vi "API - On Demand - Read 1 Digital Input Sample on Demand.vi"(8 "error in":errorcluster, 10 "Digital Input Channel Number":i32, 11 "TCP Network Connection in":refnum<k5>) -> (0 "error out":errorcluster, 2 "Boolean Data Out":bool=TRUE, 3 "TCP Network Connection out":refnum<k5>)   [LabVIEW 2020]
doc: "Read a single digital input measurement from the DAQ.\n-Enable channel\n-Start streaming of data\n-Download 1 datapoint\n-Stop streaming of data"
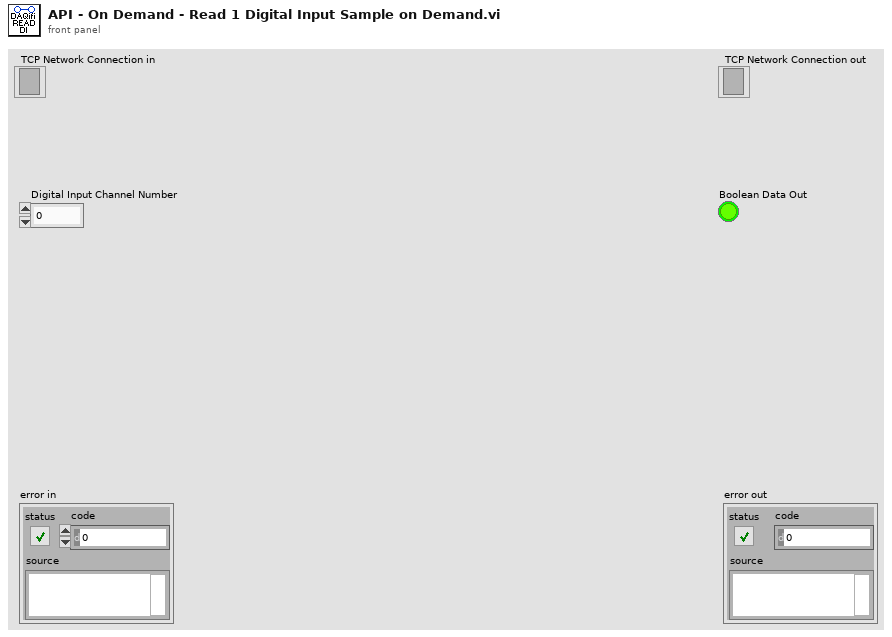
[diagram p1: front panel]
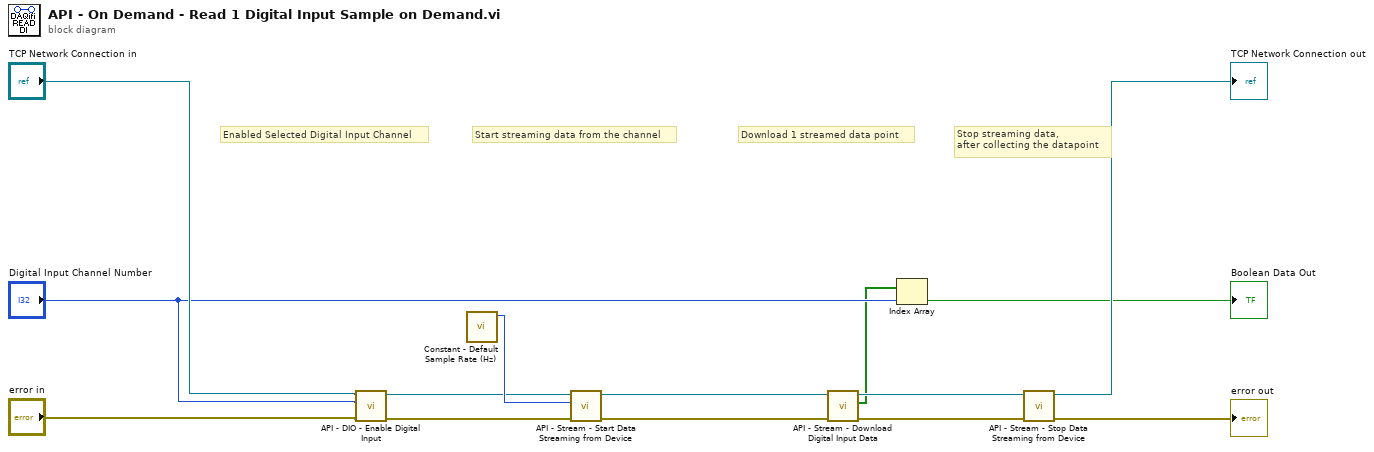
[diagram p0: block diagram]
diagram:
  # "Download 1 streamed data point"
  # "Enabled Selected Digital Input Channel"
  # "Stop streaming data,\nafter collecting the datapoint"
  # "Start streaming data from the channel"
  n1 = call "API - DIO - Enable Digital Input.vi"("error in"="error in", "Channel Number"="Digital Input Channel Number", "TCP Network Connection in"="TCP Network Connection in") -> ("error out"=w9:errorcluster, "TCP Network Connection out"=w8:refnum<k5>)  [unwired: 7 in]
  n2 = call "Constant - Default Sample Rate (Hz).vi"() -> ("Streaming Rate (Hz)"=w12:i32)  [unwired: 11 in]
  n3 = call "API - Stream - Start Data Streaming from Device.vi"("error in (no error)"=w9, "Streaming Rate (Hz)"=w12, "TCP Network Connection in"=w8) -> ("error out"=w6:errorcluster, "TCP Network Connection out"=w7:refnum<k5>)  [unwired: 7 in]
  n4 = call "API - Stream - Download Digital Input Data.vi"("error in"=w6, "TCP Network Connection in"=w7) -> ("error out"=w5:errorcluster, "Digital Inputs"=w2:bool[], "TCP Network Connection out"=w4:refnum<k5>)  [unwired: 7 in]
  n5 = Index Array(array=w2, index="Digital Input Channel Number") -> (element=→"Boolean Data Out":bool)
  n6 = call "API - Stream - Stop Data Streaming from Device.vi"("error in (no error)"=w5, "TCP Network Connection in"=w4) -> ("error out"=→"error out":errorcluster, "TCP Network Connection out"=→"TCP Network Connection out":refnum<k5>)  [unwired: 8 in]
